vi "Create Class.vi"(4 "error in":errorcluster, 6 "Class Definition":T1, 7 "Path":path) -> (0 "error out":errorcluster)   [LabVIEW 2025]
doc: "This VI creates a Class according to the provided Class definition in the specified path. This VI sets the description and the class name as defined."
uses:
  Class Definition--cluster.ctl
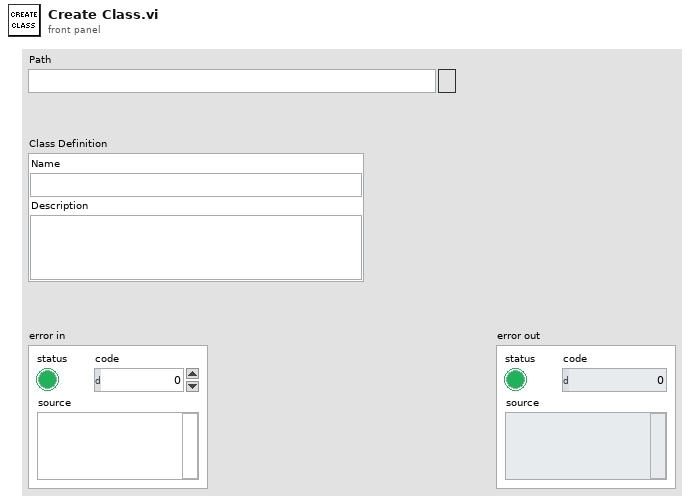
[diagram p1: front panel]
types:
  T1 = typedef "Class Definition--cluster.ctl" = cluster{"Name":string, "Description":string}
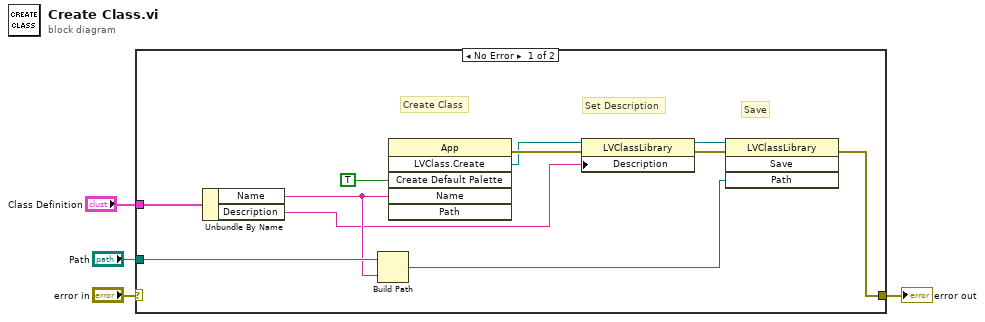
[diagram p0: block diagram]
diagram:
  n1 = case shown="No Error" "error in" {
    selector: "error in" -> [_ w16]
    tunnel: "Path" -> [w12 _]
    tunnel: "Class Definition" -> [w11 _]
    tunnel: [w15 w16] -> w3
    frame No Error {
      # "Save"
      # "Set Description"
      # "Create Class"
      n2 = Unbundle By Name(w11) -> ("Name"=w9:string, "Description"=w5:string)
      n3 = Build Path(base path=w12, name or relative path=w9) -> (appended path=w8:path)
      n4 = invoke class="App" method="LVClass.Create"("Create Default Palette"=TRUE ("Create:Default Palette"), "Name"=w9) -> (error out=w14:errorcluster, "LVClass.Create"=w6:refnum<vi>)  [unwired: 4 in, 4 out]
      n5 = property class="LVClassLibrary"(reference=w6, error in=w14, "Description"=w5) -> (reference out=w7:refnum<vi>, error out=w13:errorcluster)
      n6 = invoke class="LVClassLibrary" method="Save"(reference=w7, error in=w13, "Path"=w8) -> (error out=w15:errorcluster)  [unwired: 1 in, 3 out]
    }
    frame Error {
      # "Pass error without further action"
    }
  }
  "error out" <- w3
